vi "main.vi"() -> ()   [LabVIEW 2016]
panel:
  out "error out":errorcluster
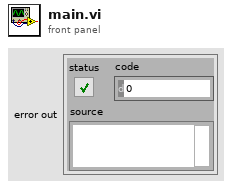
[diagram p1: front panel]
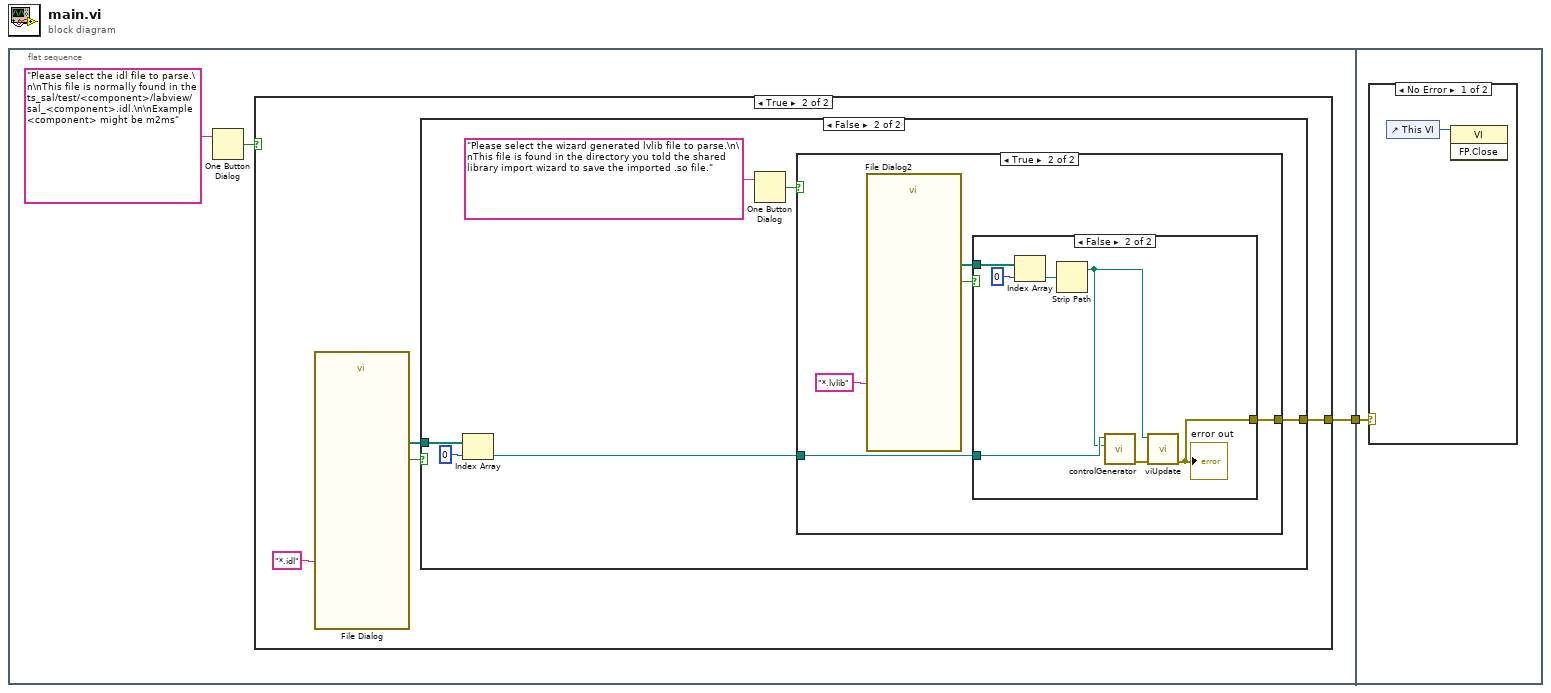
[diagram p0: block diagram]
diagram:
  n1 = flat-sequence {
    tunnel: [w2] -> w1
    tunnel: w1 -> [w27]
    frame #0 {
      n2 = One Button Dialog(message="Please select the idl file to parse.\n\nThis file is normally found in the ts_sal/test/<component>/labview/sal_<component>.idl.\n\nExample <component> might be m2ms") -> (true=w3:bool)  [unwired: 1 in]
      n3 = case shown="True" w3 {
        tunnel: [_ w5] -> w2
        frame False {
        }
        frame True {
          n4 = call "File Dialog"("pattern (all files)"="*.idl") -> ("selected paths"=w7:path[], "cancelled"=w6:bool)  [unwired: 11 in, 2 out]
          n5 = case shown="False" w6 {
            tunnel: w7 -> [_ w13]
            tunnel: [_ w9] -> w5
            frame True {
            }
            frame False {
              n6 = Index Array(array=w13, index=0) -> (element=w14:path)
              n7 = One Button Dialog(message="Please select the wizard generated lvlib file to parse.\n\nThis file is found in the directory you told the shared library import wizard to save the imported .so file.") -> (true=w10:bool)  [unwired: 1 in]
              n8 = case shown="True" w10 {
                tunnel: w14 -> [_ w17]
                tunnel: [_ w15] -> w9
                frame False {
                }
                frame True {
                  n9 = call "File Dialog2"("pattern (all files)"="*.lvlib") -> ("selected paths"=w18:path[], "cancelled"=w16:bool)  [unwired: 11 in, 2 out]
                  n10 = case shown="False" w16 {
                    tunnel: w18 -> [_ w25]
                    tunnel: w17 -> [_ w22]
                    tunnel: [_ w20] -> w15
                    frame True {
                    }
                    frame False {
                      n11 = Index Array(array=w25, index=0) -> (element=w24:path)
                      n12 = Strip Path(path=w24) -> (stripped path=w21:path)  [unwired: 1 out]
                      n13 = call "controlGenerator.vi"("ControlOutputPath"=w21, "ComponentIDLFile"=w22) -> ("error out"=w23:errorcluster)  [unwired: 9 in]
                      n14 = call "viUpdate.vi"("error in (no error)"=w23, "OutputPath"=w21) -> ("error out"=w20:errorcluster)  [unwired: 9 in]
                      "error out" <- w20
                    }
                  }
                }
              }
            }
          }
        }
      }
    }
    frame #1 {
      n15 = case shown="No Error" w27 {
        frame No Error {
          n16 = control-ref of="This VI"() -> (w28:refnum<vi>)
          n17 = invoke class="VI" method="FP.Close"(reference=w28) -> ()  [unwired: 2 in, 3 out]
        }
        frame Error {
        }
      }
    }
  }
